vi "Offline_Analysis_FLDA_분석기.vi"(0 "LDA_matrix":path caption="LDA_matrix.txt", 5 "Weight":path caption="weight.txt", 7 "Target_order.txt":path, 9 "mius_flash_order":path, 11 "Brain":path, 12 "피험자이름":string="홍길동", 13 "Save_path":string="Emotion_Research\\Result") -> ()   [LabVIEW 2014]
uses:
  <vilib>/Utility/file.llb/Read From Spreadsheet File (DBL).vi
  <vilib>/Analysis/Matrix/Numeric/Conversions/Array To Matrix - RA2.vi
  <vilib>/Analysis/Matrix/Numeric/Conversions/Array To Matrix - RA.vi
  <vilib>/Utility/file.llb/Read From Spreadsheet File (I64).vi
  <vilib>/Utility/file.llb/Write To Spreadsheet File (DBL).vi
  <vilib>/Utility/file.llb/Write To Spreadsheet File (I64).vi
  <vilib>/Utility/file.llb/Write To Spreadsheet File (string).vi
  <vilib>/Analysis/Matrix/NI_Matrix.lvlib
panel:
  out "ACC":i16
  in  "Channel selection":bool[](array[boolean])=[TRUE, TRUE, TRUE, TRUE, TRUE, TRUE, TRUE, TRUE, TRUE, TRUE, TRUE]
  out "Target_order":i64[](array[numeric])
  out "Selected_Target":i32[](array[numeric])
  out "Accuracy":i16[](array[numeric])
  in  "사용할 Parameter 갯수":i32=4
  out "error out":errorcluster
  in  "Random_num":i32=6
  in  "Flash_Repeat":i32=20
  in  "Frame_Length":i32=10
  in  "Sampling_Rate":dbl=512.0
  in  "ERP_Parameters_of_NonTarget":path caption="ERP_Parameters_of_NonTarget.txt"
  in  "ERP_Parameters_of_Target":path caption="ERP_Parameters_of_Target.txt"
  # "ERP_Parameter안씀. LDA바로 집어넣으면 됨"
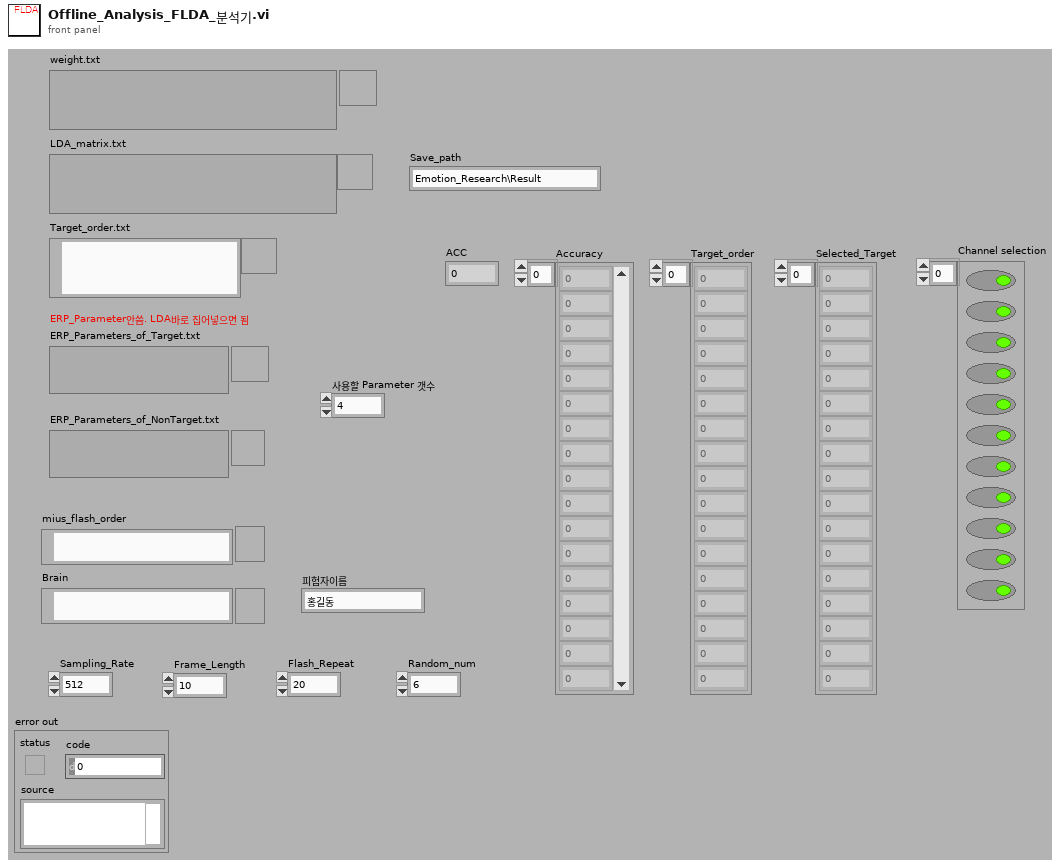
[diagram p1: front panel]
types:
  T1 = typedef "NI_Matrix.lvlib/RealMatrix.ctl" = dbl[][]
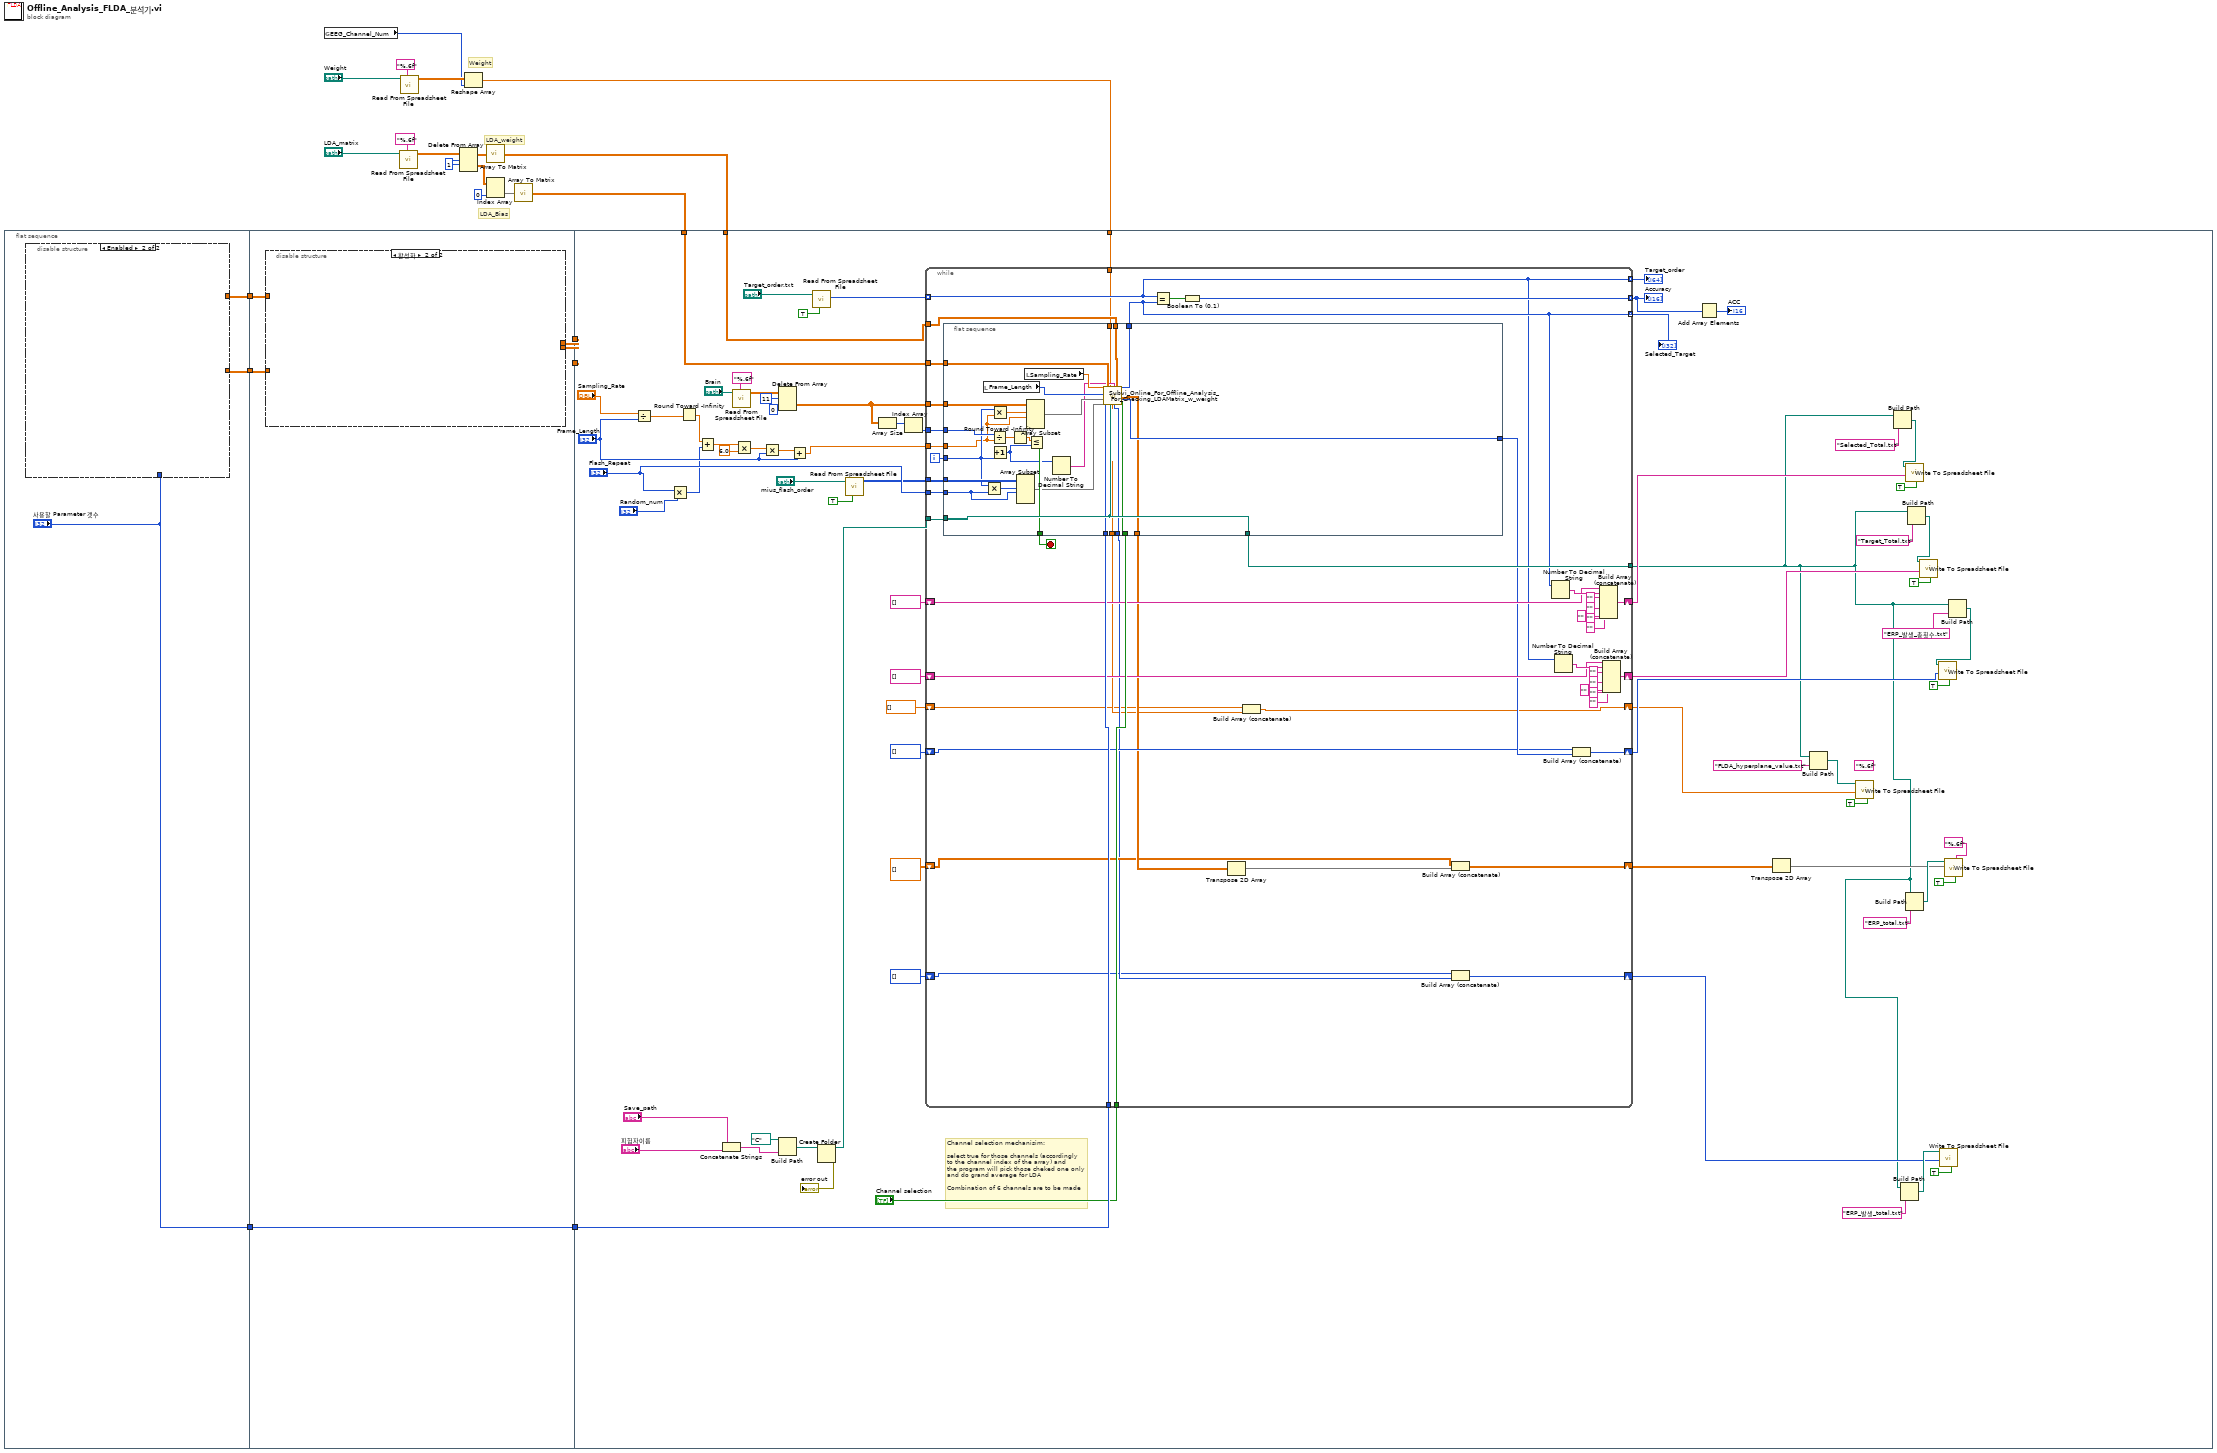
[diagram p0: block diagram]
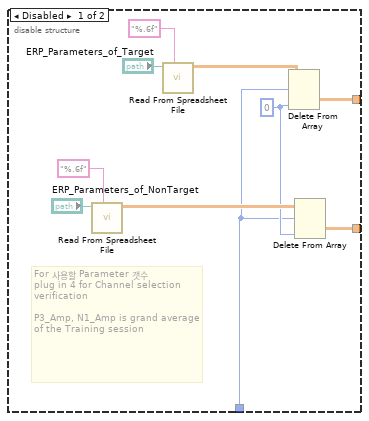
[diagram p2: hidden frame]
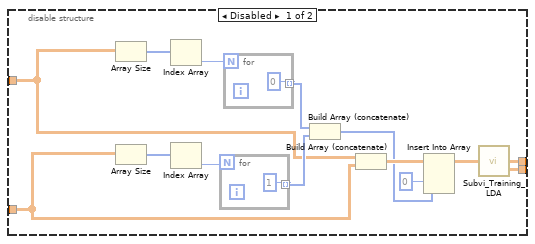
[diagram p3: hidden frame]
diagram:
  w10 = 1 ("인덱스 (행)")
  # "LDA_Bias"
  # "LDA_weight"
  # "Weight"
  n1 = flat-sequence {
    tunnel: [w24] -> w21
    tunnel: [w23] -> w20
    tunnel: ["사용할 Parameter 갯수"] -> w17
    tunnel: w21 -> [w39]
    tunnel: w20 -> [w38]
    tunnel: [w37] -> w19
    tunnel: [w36] -> w18
    tunnel: w17 -> [w35]
    tunnel: [w35] -> w16
    tunnel: w19 -> [_]
    tunnel: w18 -> [_]
    tunnel: w16 -> [w104]
    tunnel: w7 -> [w68]
    tunnel: w6 -> [w67]
    tunnel: w1 -> [w66]
    frame #0 {
      n2 = disable-structure shown="Enabled" {
        disable-tunnel: [w27 _] -> w24
        disable-tunnel: [w26 _] -> w23
        disable-tunnel: "사용할 Parameter 갯수" -> [w25 _]
        frame Disabled {
          w28 = 0 ("비활성화된 인덱스 (열)")
          # "For 사용할 Parameter 갯수\nplug in 4 for Channel selection\nverification\n\nP3_Amp, N1_Amp is grand average of the Training session"
          n3 = call-poly <vilib>:"Read From Spreadsheet File.vi"("format (%.3f)"="%.6f", "file path (dialog if empty)"="ERP_Parameters_of_NonTarget") -> ("all rows"=w29:dbl[][])  [unwired: 5 in, 4 out]
          n4 = call-poly <vilib>:"Read From Spreadsheet File.vi"("format (%.3f)"="%.6f", "file path (dialog if empty)"="ERP_Parameters_of_Target") -> ("all rows"=w30:dbl[][])  [unwired: 5 in, 4 out]
          n5 = Delete From Array(array=w30, length=w25, index (col)=w28) -> (deleted portion=w27:dbl[][])  [unwired: 1 in, 1 out]
          n6 = Delete From Array(array=w29, length=w25, index (col)=w28) -> (deleted portion=w26:dbl[][])  [unwired: 1 in, 1 out]
        }
        frame Enabled {
        }
      }
    }
    frame #1 {
      n7 = disable-structure shown="활성화" {
        disable-tunnel: w39 -> [w44 _]
        disable-tunnel: w38 -> [w43 _]
        disable-tunnel: [w42 _] -> w37
        disable-tunnel: [w41 _] -> w36
        frame Disabled {
          n8 = Array Size(array=w44) -> (size(s)=w48:i32[])
          n9 = Array Size(array=w43) -> (size(s)=w49:i32[])
          n10 = Index Array(array=w48) -> (element=w50:i32)  [unwired: 1 in]
          n11 = Index Array(array=w49) -> (element=w51:i32)  [unwired: 1 in]
          n12 = for {
            N: w51 -> [_]
            tunnel: [1] -> w53 mode=indexing
          }
          n13 = for {
            N: w50 -> [_]
            tunnel: [0] -> w52 mode=indexing
          }
          n14 = Build Array (concatenate)(w52, w53) -> (w45:i32[])
          n15 = Build Array (concatenate)(w44, w43) -> (w46:dbl[][])
          n16 = Insert Into Array(array=w46, index (col)=0 ("비활성화된 인덱스 (열)"), new element=w45) -> (w40:dbl[][])  [unwired: 1 in]
          n17 = call "Subvi_Training_LDA.vi"("Input_Data"=w40) -> ("A * B 2"=w42:T1, "A * B"=w41:T1)
        }
        frame Enabled {
        }
      }
    }
    frame #2 {
      (unwired) "%.6f" ("format (%.3f)")
      # "Channel selection mechanisim:\n\nselect true for those channels (accordingly\nto the channel index of the array) and \nthe program will pick those cheked one only\nand do grand average for LDA\n\nCombination of 6 channels are to be made"
      n18 = Divide(x="Sampling_Rate", y="Frame_Length") -> (x/y=w114:dbl)
      n19 = Multiply(x="Flash_Repeat", y="Random_num") -> (x*y=w117:i32)
      n20 = Round Toward -Infinity(1:w114) -> (0:w116:dbl)
      n21 = Add(x=w116, y=w117) -> (x+y=w119:dbl)
      n22 = Concatenate Strings("Save_path", "피험자이름") -> (w59:string)
      n23 = call-poly <vilib>:"Read From Spreadsheet File.vi"("format (%.3f)"="%.6f", "file path (dialog if empty)"="Brain") -> ("all rows"=w57:dbl[][])  [unwired: 5 in, 4 out]
      n24 = Multiply(x=w119, y=6.0) -> (x*y=w121:dbl)
      n25 = Multiply(x=w121, y="Frame_Length") -> (x*y=w123:dbl)
      n26 = Build Path(base path=path "C:/" ("path"), name or relative path=w59) -> (appended path=w126:path)
      n27 = Delete From Array(array=w57, length=11 ("길이"), index (col)=0 ("비활성화된 인덱스 (열)")) -> (deleted portion=w56:dbl[][])  [unwired: 1 in, 1 out]
      n28 = Add(x=w123, y="Frame_Length") -> (x+y=w124:dbl)
      n29 = call-poly <vilib>:"Read From Spreadsheet File.vi"("transpose (no:F)"=TRUE, "file path (dialog if empty)"="Target_order.txt") -> ("first row"=w102:i64[])  [unwired: 5 in, 4 out]
      n30 = Create Folder(path (use dialog)=w126) -> (created path=w128:path, error out=→"error out":errorcluster)  [unwired: 2 in, 1 out]
      n31 = call-poly <vilib>:"Read From Spreadsheet File.vi"("transpose (no:F)"=TRUE, "file path (dialog if empty)"="mius_flash_order") -> ("all rows"=w110:i64[][])  [unwired: 5 in, 4 out]
      n32 = Array Size(array=w56) -> (size(s)=w111:i32[])
      n33 = Index Array(array=w111) -> (element=w112:i32)  [unwired: 1 in]
      n34 = while {
        tunnel: w67 -> [w177]
        tunnel: w68 -> [w176]
        tunnel: w56 -> [w174]
        tunnel: w110 -> [w173]
        tunnel: w112 -> [w175]
        tunnel: w124 -> [w171]
        tunnel: "Flash_Repeat" -> [w172]
        tunnel: w128 -> [w170]
        tunnel: w104 -> [w169]
        tunnel: w102 -> [w147] mode=indexing
        tunnel: [w167] -> w90 mode=indexing
        tunnel: [w147] -> w99 mode=indexing
        tunnel: [w148] -> w100 mode=indexing
        tunnel: "Channel selection" -> [w164]
        tunnel: [w163] -> w61
        shift-right: [w150] -> w84
        shift-left: string[] [] -> [w149]
        shift-right: [w146] -> w83
        shift-left: string[] [] -> [w145]
        shift-right: [w143] -> w81
        shift-left: i16[] [] -> [w142]
        shift-right: [w139] -> w76
        shift-left: dbl[][] [] -> [w138]
        shift-right: [w136] -> w69
        shift-left: i16[] [] -> [w135]
        tunnel: w66 -> [w134]
        shift-right: [w131] -> w60
        shift-left: dbl[] [] -> [w132]
        i -> [w166]
        stop <- w165 stop-if-true
        n35 = flat-sequence {
          tunnel: [w205] -> w144
          tunnel: [w204] -> w163
          tunnel: w134 -> [w180]
          tunnel: [w181] -> w137
          tunnel: [w183] -> w141
          tunnel: w164 -> [w184]
          tunnel: [w185] -> w148
          tunnel: w169 -> [w186]
          tunnel: w170 -> [w204]
          tunnel: w171 -> [w192]
          tunnel: w166 -> [w193]
          tunnel: w172 -> [w194]
          tunnel: w173 -> [w196]
          tunnel: w174 -> [w199]
          tunnel: [w200] -> w165
          tunnel: w175 -> [w201]
          tunnel: w176 -> [w202]
          tunnel: w177 -> [w203]
          tunnel: [w178] -> w133
          frame #0 {
            n36 = local read "Frame_Length"() -> (w188:i32)
            n37 = Multiply(x=w193, y=w194) -> (x*y=w195:i32)
            n38 = Divide(x=w201, y=w192) -> (x/y=w191:dbl)
            n39 = Multiply(x=w193, y=w192) -> (x*y=w198:dbl)
            n40 = Increment(x=w193) -> (x+1=w187:i32)
            n41 = Round Toward -Infinity(1:w191) -> (0:w190:dbl)
            n42 = Array Subset(array=w196, index (row)=w195, length (row)=w194) -> (w179:i64[][])  [unwired: 2 in]
            n43 = local read "Sampling_Rate"() -> (w189:dbl)
            n44 = Array Subset(array=w199, index (row)=w198, length (row)=w192) -> (w197:dbl[][])  [unwired: 2 in]
            n45 = Less Or Equal?(x=w190, y=w187) -> (x <= y?=w200:bool)
            n46 = Number To Decimal String(number=w187) -> (decimal integer string=w182:string)  [unwired: 1 in]
            n47 = call "Subvi_Online_For_Offline_Analysis_For_Checking_LDAMatrix_w_weight.vi"("rate"=w189, "samples per channel"=w188, "Brain_data_source"=w197, "Target_Flash_Order"=w179, "Value"=w203, "사용할 Parameter 갯수"=w186, "Weight"=w180, "Path"=w204, "Number"=w182, "Matrix"=w202, "Channel selection"=w184) -> ("Array"=w178:dbl[], "자극별 ERP 발생여부"=w181:i16[], "output-0~8"=w185:i32, "ERP_all"=w183:dbl[][], "자극별 ERP 발생 총 횟수"=w205:i16[])  [unwired: 12 in]
          }
        }
        n48 = Equal?(x=w147, y=w148) -> (x = y?=w168:bool)
        n49 = Boolean To (0,1)(Boolean=w168) -> (0, 1=w167:i16)
        n50 = Transpose 2D Array(2D array=w141) -> (transposed array=w140:dbl[][])
        n51 = Build Array (concatenate)(w132, w133) -> (w131:dbl[])
        n52 = Build Array (concatenate)(w135, w137) -> (w136:i16[])
        n53 = Build Array (concatenate)(w138, w140) -> (w139:dbl[][])
        n54 = Number To Decimal String(number=w148) -> (decimal integer string=w156:string)  [unwired: 1 in]
        n55 = Number To Decimal String(number=w147) -> (decimal integer string=w162:string)  [unwired: 1 in]
        n56 = Build Array (concatenate)(w142, w144) -> (w143:i16[])
        n57 = Build Array (concatenate)(w149, w156, "" ("element"), "" ("element"), "" ("element"), "" ("element"), "" ("element")) -> (w150:string[])
        n58 = Build Array (concatenate)(w145, w162, "" ("element"), "" ("element"), "" ("element"), "" ("element"), "" ("element")) -> (w146:string[])
      }
      "Accuracy" <- w90
      "Selected_Target" <- w100
      "Target_order" <- w99
      n59 = Add Array Elements(numeric array=w90) -> (sum=→"ACC":i16)
      n60 = Transpose 2D Array(2D array=w76) -> (transposed array=w74:dbl[][])
      n61 = Build Path(base path=w61, name or relative path="FLDA_hyperplane_value.txt") -> (appended path=w63:path)
      n62 = call-poly <vilib>:"Write To Spreadsheet File.vi"("transpose? (no:F)"=TRUE, "1D data"=w60, "file path (dialog if empty)"=w63) -> ()  [unwired: 5 in, 1 out]
      n63 = Build Path(base path=w61, name or relative path="Selected_Total.txt") -> (appended path=w86:path)
      n64 = Build Path(base path=w61, name or relative path="ERP_발생_total.txt") -> (appended path=w71:path)
      n65 = call-poly <vilib>:"Write To Spreadsheet File.vi"("transpose? (no:F)"=TRUE, "1D data"=w84, "file path (dialog if empty)"=w86) -> ()  [unwired: 5 in, 1 out]
      n66 = Build Path(base path=w61, name or relative path="ERP_total.txt") -> (appended path=w77:path)
      n67 = Build Path(base path=w61, name or relative path="Target_Total.txt") -> (appended path=w92:path)
      n68 = call-poly <vilib>:"Write To Spreadsheet File.vi"("transpose? (no:F)"=TRUE, "1D data"=w83, "file path (dialog if empty)"=w92) -> ()  [unwired: 5 in, 1 out]
      n69 = call-poly <vilib>:"Write To Spreadsheet File.vi"("transpose? (no:F)"=TRUE, "1D data"=w69, "file path (dialog if empty)"=w71) -> ()  [unwired: 5 in, 1 out]
      n70 = call-poly <vilib>:"Write To Spreadsheet File.vi"("transpose? (no:F)"=TRUE, "format (%.3f)"="%.6f", "2D data"=w74, "file path (dialog if empty)"=w77) -> ()  [unwired: 4 in, 1 out]
      n71 = Build Path(base path=w61, name or relative path="ERP_발생_총횟수.txt") -> (appended path=w94:path)
      n72 = call-poly <vilib>:"Write To Spreadsheet File.vi"("transpose? (no:F)"=TRUE, "1D data"=w81, "file path (dialog if empty)"=w94) -> ()  [unwired: 5 in, 1 out]
    }
  }
  n73 = global read "Control_Panel_정리.vi" "EEG_Channel_Num"() -> (w2:i32)
  n74 = call-poly <vilib>:"Read From Spreadsheet File.vi"("format (%.3f)"="%.6f", "file path (dialog if empty)"="LDA_matrix") -> ("all rows"=w8:dbl[][])  [unwired: 5 in, 4 out]
  n75 = call-poly <vilib>:"Read From Spreadsheet File.vi"("format (%.3f)"="%.6f", "file path (dialog if empty)"="Weight") -> ("all rows"=w3:dbl[][])  [unwired: 5 in, 4 out]
  n76 = Delete From Array(array=w8, length=w10, index (row)=w10) -> (deleted portion=w13:dbl[][], array with subset deleted=w12:dbl[][])  [unwired: 1 in]
  n77 = Reshape Array(w3, w2) -> (w1:dbl[])
  n78 = call-poly <vilib>:"Array To Matrix.vi"("Real 2D Array"=w12) -> ("Real Matrix"=w7:T1)
  n79 = Index Array(array=w13, index (col)=0 ("인덱스")) -> (element=w11:dbl[])  [unwired: 1 in]
  n80 = call-poly <vilib>:"Array To Matrix.vi"("Real 1D Array"=w11) -> ("Real Matrix (Column Vector)"=w6:T1)
